vi "Configure Acquisition.vi"(8 "error in":errorcluster, 11 "HDO4000A Base CFG in":refnum<class "HDO4000A Base CFG.lvclass">) -> (0 "error out":errorcluster, 3 "HDO4000A Base CFG out":refnum<class "HDO4000A Base CFG.lvclass">)   [LabVIEW 2023, in "HDO4000A Base CFG.lvclass"]
uses:
  HDO4000A Base CFG.lvclass
  HDO4000A Base CFG.lvclass/HDO4000A Base CFG.ctl
  HAL/Configuration Base/Configuration Base.lvclass
  b866a249-2c16-4da1-b915-f131202624c1.vi
  6eb31647-1959-4f32-b65e-888234ee7fb3.vi
  <vilib>/Utility/error.llb/Error Cluster From Error Code.vi
  <vilib>/ErrorRing/Error Ring.xnode
  ca641a30-c0a1-4d05-a20f-987cfa858d1a.vi
  HAL/Scope VISA/Configuration/Scope VISA CFG.lvclass
  D:/git/HAL/Scope VISA/Configuration/Scope VISA CFG.lvclass
  D:/git/HAL/Configuration Base/Configuration Base.lvclass
  D:/git/HAL/Interfaces/IConfigure/IConfigure.lvclass
  D:/git/HAL/Interfaces/IConfigure Scope/IConfigure Scope.lvclass
  D:/git/LeCroy-HDO4000A-LabVIEW/Configurations/HDO4000A Base CFG/HDO4000A Base CFG.lvclass
  <instrlib>/LeCroy Wave Series/LeCroy Wave Series.lvlib
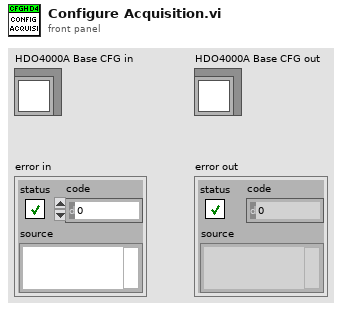
[diagram p1: front panel]
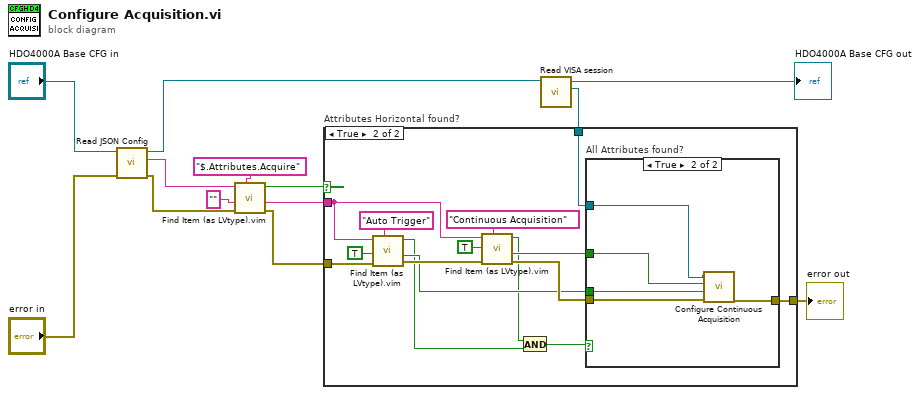
[diagram p0: block diagram]
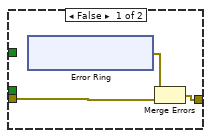
[diagram p3: hidden frame]
diagram:
  n1 = call "Read JSON Config.vi"("error in (no error)"="error in", "object in"="HDO4000A Base CFG in") -> ("error out"=w10:errorcluster, "<JSON>Config"=w9:string, "object out"=w3:refnum<class "HDO4000A Base CFG.lvclass">)  [unwired: 7 in]
  n2 = call "Find Item (as LVtype).vim"("$Path or Item Name"="$.Attributes.Acquire", "error in (no error)"=w10, "Data Type and Default Value"="", "JSON"=w9) -> ("error out"=w6:errorcluster, "Data"=w7:string, "Found"=w8:bool)  [unwired: 4 in, 1 out]
  n3 = call "Read VISA session.vi"("Scope VISA CFG in"=w3) -> ("VISA session"=w2:refnum<visa-resource-name>, "Scope VISA CFG out"=→"HDO4000A Base CFG out":refnum<class "HDO4000A Base CFG.lvclass">)  [unwired: 8 in, 1 out]
  n4 = case "Attributes Horizontal found?" shown="True" w8 {
    tunnel: w7 -> [_ w23]
    tunnel: w6 -> [w14 w22]
    tunnel: w2 -> [_ w27]
    tunnel: [w14 w16] -> w1
    frame False {
    }
    frame True {
      n5 = call "Find Item (as LVtype).vim"("$Path or Item Name"="Auto Trigger", "error in (no error)"=w22, "Data Type and Default Value"=TRUE, "JSON"=w23) -> ("error out"=w21:errorcluster, "Data"=w19:bool, "Found"=w18:bool)  [unwired: 4 in, 1 out]
      n6 = call "Find Item (as LVtype).vim"("$Path or Item Name"="Continuous Acquisition", "error in (no error)"=w21, "Data Type and Default Value"=TRUE, "JSON"=w23) -> ("error out"=w20:errorcluster, "Data"=w26:bool, "Found"=w17:bool)  [unwired: 4 in, 1 out]
      n7 = And(x=w17, y=w18) -> (x .and. y?=w15:bool)
      n8 = case "All Attributes found?" shown="True" w15 {
        tunnel: w27 -> [_ w41]
        tunnel: w26 -> [_ w39]
        tunnel: w20 -> [w31 w40]
        tunnel: w19 -> [_ w38]
        tunnel: [w30 w42] -> w16
        frame False {
          n9 = xnode "Error Ring"() -> ("error out"=w32:errorcluster)
          n10 = Merge Errors(w32, w31) -> (w30:errorcluster)
        }
        frame True {
          n11 = call <instrlib>:"Configure Continuous Acquisition.vi"("error in (no error)"=w40, "Auto Trigger Enabled (T: Normal)"=w38, "Continuous Acquisition Mode (T: On)"=w39, "VISA resource name"=w41) -> ("error out"=w42:errorcluster)  [unwired: 6 in, 1 out]
        }
      }
    }
  }
  "error out" <- w1
